vi "Target Send to Logging.vi"(6 "rt fifo":refnum<k33>, 11 "Target Sensors":T1) -> ()   [LabVIEW 2018]
uses:
  Ankle Benchtop Testing Advanced/Target Sensors.ctl
  Ankle Benchtop Testing Advanced/Target Raw Sensors.ctl
  Ankle Benchtop Testing Advanced/Target Filtered Sensors.ctl
  Ankle Benchtop Testing Advanced/Target Logging Cluster.ctl
  COBRA Logging and Loop Timing Library.lvlib
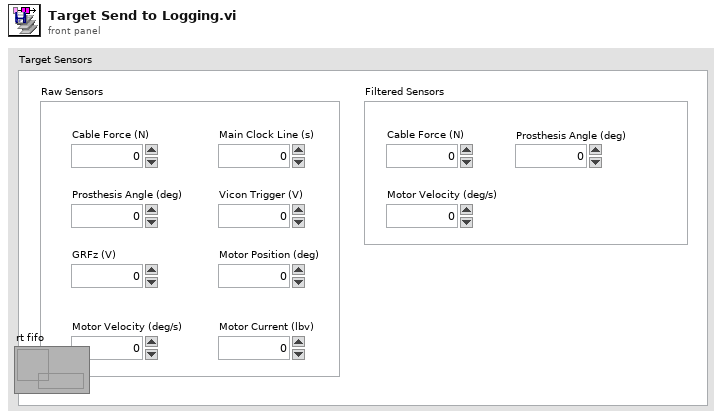
[diagram p1: front panel]
types:
  T1 = typedef "Target Sensors.ctl" = cluster{"Raw Sensors":T2, "Filtered Sensors":T3}
  T2 = typedef "Target Raw Sensors.ctl" = cluster{"Cable Force (N)":dbl, "Prosthesis Angle (deg)":dbl, "Main Clock Line (s)":dbl, "Vicon Trigger (V)":dbl, "GRFz (V)":dbl, "Motor Position (deg)":dbl, "Motor Velocity (deg/s)":dbl, "Motor Current (lbv)":dbl}
  T3 = typedef "Target Filtered Sensors.ctl" = cluster{"Cable Force (N)":dbl, "Prosthesis Angle (deg)":dbl, "Motor Velocity (deg/s)":dbl}
  T4 = typedef "Target Logging Cluster.ctl" = cluster{"Valid for Logging?":bool, "Target Sensors":T1}
  T5 = enum16{"Manual Button Press", "External Voltage"}
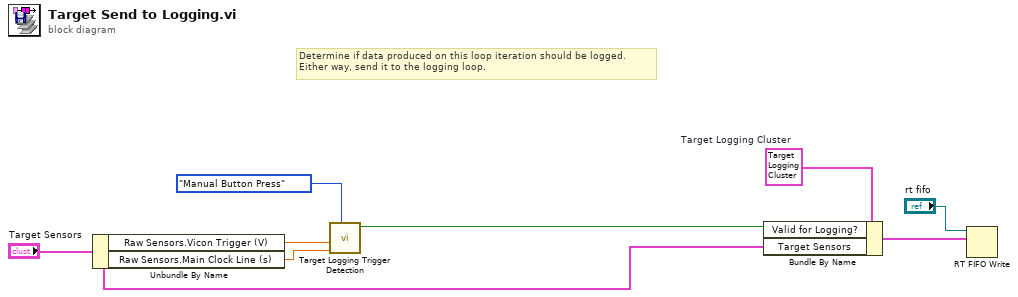
[diagram p0: block diagram]
diagram:
  w6 = T4 {"Valid for Logging?"=FALSE, "Target Sensors"={"Raw Sensors"={"Cable Force (N)"=0.0, "Prosthesis Angle (deg)"=0.0, "Main Clock Line (s)"=0.0, "Vicon Trigger (V)"=0.0, "GRFz (V)"=0.0, "Motor Position (deg)"=0.0, "Motor Velocity (deg/s)"=0.0, "Motor Current (lbv)"=0.0}, "Filtered Sensors"={"Cable Force (N)"=0.0, "Prosthesis Angle (deg)"=0.0, "Motor Velocity (deg/s)"=0.0}}}  # Target Logging Cluster
  # "Determine if data produced on this loop iteration should be logged.\nEither way, send it to the logging loop."
  n1 = Unbundle By Name("Target Sensors") -> ("Raw Sensors.Vicon Trigger (V)"=w3:dbl, "Raw Sensors.Main Clock Line (s)"=w2:dbl)
  n2 = call "Target Logging Trigger Detection.vi"("Trigger Mode"=T5."Manual Button Press", "Main Clock Line (s)"=w2, "External Trigger Voltage"=w3) -> ("Valid for Logging?"=w4:bool)  [unwired: 8 in]
  n3 = Bundle By Name(cluster=w6, "Valid for Logging?"=w4, "Target Sensors"="Target Sensors") -> (w7:T4)
  n4 = RT FIFO Write(0:"rt fifo", 1:w7) -> ()  [unwired: 3 in, 4 out]
